vi "Create.vi"(8 "error in (no error)":errorcluster, 11 "Actor in":refnum<class "Copy of Actor.lvclass">) -> (0 "error out":errorcluster, 3 "API-Reference out":refnum<k1>)   [LabVIEW 2018, in "Copy of Actor.lvclass"]
uses:
  Copy of Actor.lvclass
  API-Data.ctl
  Stopped.ctl
  Event-References.ctl
  Stop.ctl
  Launched.ctl
  Some Request.ctl
  Some Response.ctl
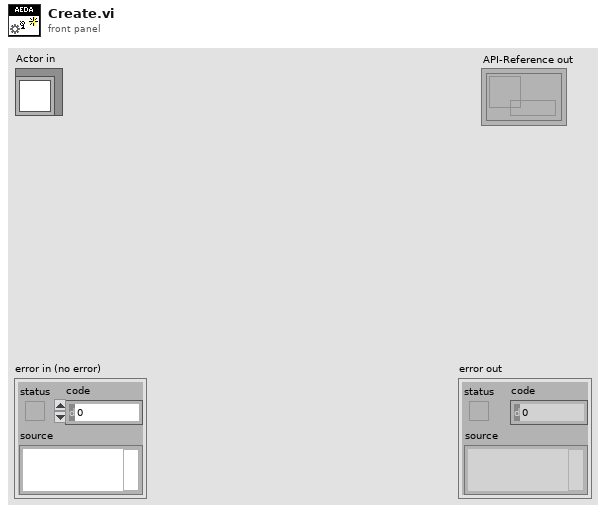
[diagram p1: front panel]
types:
  T1 = typedef "Copy of Actor.lvclass/Event-References.ctl" = cluster{"Stop":refnum<user-event>, "Launched":refnum<user-event>, "Some Request":refnum<user-event>}
  T2 = typedef "Copy of Actor.lvclass/Stopped.ctl" = cluster{"Final State":refnum<class "Copy of Actor.lvclass">, "Final Error":errorcluster}
  T3 = typedef "Copy of Actor.lvclass/API-Data.ctl" = cluster{"Launch":refnum<notifier>, "Stopped":refnum<user-event>, "Actor-Events":T1, "Stopped Registration":refnum<event-registration>}
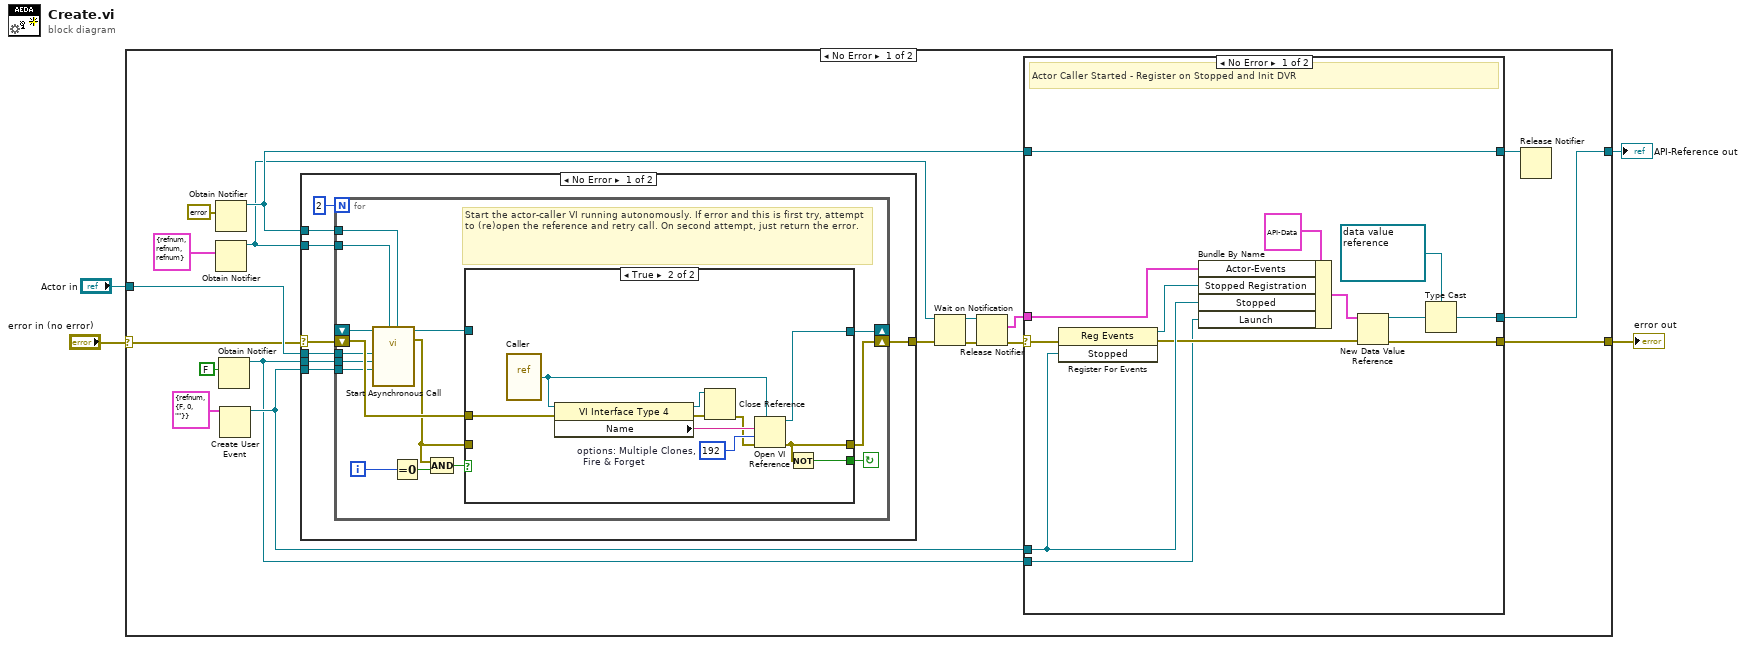
[diagram p0: block diagram]
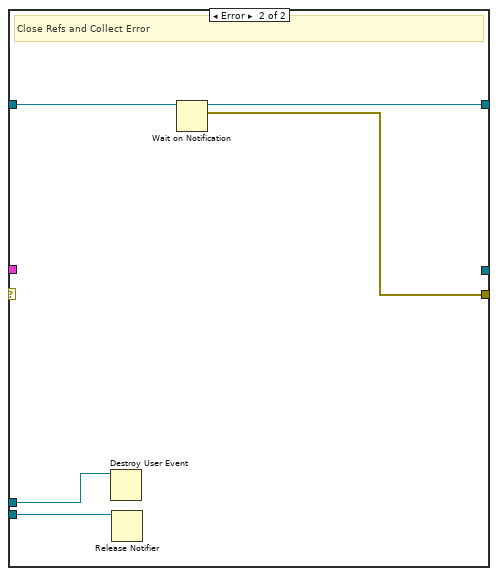
[diagram p4: hidden frame]
diagram:
  n1 = case shown="No Error" "error in (no error)" {
    selector: "error in (no error)" -> [w7 w77]
    tunnel: [w20 w77] -> w3
    tunnel: "Actor in" -> [w15 _]
    tunnel: [w19 _] -> w1
    frame No Error {
      n2 = Obtain Notifier(notification data type=errorcluster {"status"=FALSE, "code"=0, "source"=""} ("error constant")) -> (notifier out=w16:refnum<notifier>)  [unwired: 3 in, 2 out]
      n3 = Obtain Notifier(notification data type=T1 {"Stop"=refnum, "Launched"=refnum, "Some Request"=refnum} ("Actor-Events")) -> (notifier out=w12:refnum<notifier>)  [unwired: 3 in, 2 out]
      n4 = Obtain Notifier(notification data type=FALSE ("Launch")) -> (notifier out=w5:refnum<notifier>)  [unwired: 3 in, 2 out]
      n5 = Create User Event(user event datatype=T2 {"Final State"=refnum, "Final Error"={"status"=FALSE, "code"=0, "source"=""}} ("Stopped")) -> (user event=w6:refnum<user-event>)  [unwired: 1 in, 1 out]
      n6 = case shown="No Error" w7 {
        selector: w7 -> [w28 w58]
        tunnel: [w29 w58] -> w14
        tunnel: w12 -> [w27 _]
        tunnel: w16 -> [w26 _]
        tunnel: w15 -> [w25 _]
        tunnel: w5 -> [w24 _]
        tunnel: w6 -> [w23 _]
        frame No Error {
          n7 = for {
            N: 2 -> [_]
            shift-right: [w45] -> w29
            shift-left: w28 -> [w40]
            shift-right: [w39] -> _
            shift-left: _ -> [w38]
            tunnel: w27 -> [w31]
            tunnel: w26 -> [w35]
            tunnel: w25 -> [w34]
            tunnel: w24 -> [w33]
            tunnel: w23 -> [w32]
            i -> [w42]
            stop <- w41 continue-if-true
            # "Start the actor-caller VI running autonomously. If error and this is first try, attempt to (re)open the reference and retry call. On second attempt, just return the error."
            n8 = call-by-ref "Start Asynchronous Call"(reference=w38, "Initialize-Error Passback"=w35, "Events Passback"=w31, "Stopped Event"=w32, "Launch"=w33, "Actor in"=w34) -> (reference out=w37:refnum<vi>, error out=w36:errorcluster)  [unwired: 8 in]
            n9 = Equal To 0?(x=w42) -> (x = 0?=w43:bool)
            n10 = Compound Arithmetic op=AND(w36, w43) -> (w44:bool)
            n11 = case shown="True" w44 {
              tunnel: [w46 w54] -> w39
              tunnel: [w47 w56] -> w45
              tunnel: w36 -> [w47 _]
              tunnel: [_ w57] -> w41
              tunnel: w40 -> [_ w55]
              tunnel: w37 -> [w46 _]
              frame False {
              }
              frame True {
                w52 = 192  # options: Multiple Clones,   Fire & Forget
                n12 = vi-ref "Caller.vi"() -> (w48:refnum<vi>)
                n13 = property class="VI Interface Type 4"(reference=w48, error in=w55) -> (reference out=w50:refnum<vi>, error out=w51:errorcluster, "Name"=w53:string)
                n14 = Close Reference(reference=w50, error in (no error)=w51) -> (error out=w49:errorcluster)
                n15 = Open VI Reference(type specifier VI Refnum (for type only)=w48, vi path=w53, options=w52, error in (no error)=w49) -> (vi reference=w54:refnum<vi>, error out=w56:errorcluster)  [unwired: 2 in]
                n16 = Not(x=w56) -> (.not. x?=w57:bool)
              }
            }
          }
        }
        frame Error {
        }
      }
      n17 = Wait on Notification(notifier=w12, error in (no error)=w14) -> (notifier out=w11:refnum<notifier>, error out=w10:errorcluster)  [unwired: 2 in, 2 out]
      n18 = Release Notifier(notifier=w11, error in (no error)=w10) -> (last notification=w8:T1, error out=w9:errorcluster)  [unwired: 1 in, 1 out]
      n19 = case shown="No Error" w9 {
        selector: w9 -> [w67 _]
        tunnel: w8 -> [w68 _]
        tunnel: w16 -> [w71 w76]
        tunnel: [w71 w75] -> w21
        tunnel: [w69 w74] -> w20
        tunnel: [w61 _] -> w19
        tunnel: w6 -> [w65 w73]
        tunnel: w5 -> [w63 w72]
        frame No Error {
          # "Actor Caller Started - Register on Stopped and Init DVR"
          n20 = register-events(error in=w67, w65) -> (reference out=w66:refnum<event-registration>, error out=w64:errorcluster)  [unwired: 1 in]
          n21 = Bundle By Name(cluster=T3 {"Launch"=refnum, "Stopped"=refnum, "Actor-Events"={"Stop"=refnum, "Launched"=refnum, "Some Request"=refnum}, "Stopped Registration"=refnum} ("API-Data"), "Actor-Events"=w68, "Stopped Registration"=w66, "Stopped"=w65, "Launch"=w63) -> (w70:T3)
          n22 = New Data Value Reference(data value=w70, error in=w64) -> (data value reference=w62:refnum<data-value>, error out=w69:errorcluster)
          n23 = Type Cast(type=refnum<k1> refnum ("API-Reference out"), x=w62) -> (*(type *) &x=w61:refnum<k1>)
        }
        frame Error {
          # "Close Refs and Collect Error"
          n24 = Destroy User Event(user event=w73) -> ()  [unwired: 1 in, 1 out]
          n25 = Release Notifier(notifier=w72) -> ()  [unwired: 2 in, 3 out]
          n26 = Wait on Notification(notifier=w76) -> (notifier out=w75:refnum<notifier>, notification=w74:errorcluster)  [unwired: 3 in, 2 out]
        }
      }
      n27 = Release Notifier(notifier=w21) -> ()  [unwired: 2 in, 3 out]
    }
    frame Error {
    }
  }
  "error out" <- w3
  "API-Reference out" <- w1
